vi "Calculate Dispersion.vi"(5 "grating index (current)":i8=-1, 7 "turret index (0)":u8, 8 "error in (no error)":errorcluster, 10 "wavelength, nm (current)":dbl=-1.0, 11 "SOL MS in":refnum<class "PL SOL Instruments MS.lvclass">) -> (0 "error out":errorcluster, 2 "dispersion, nm/mm":dbl, 3 "SOL MS out":refnum<class "PL SOL Instruments MS.lvclass">)   [LabVIEW 2015, in "PL SOL Instruments MS.lvclass"]
doc: "Calculates <b>dispersion</b> at the specified <b>wavelength</b> for the specified <b>grating</b> of the specified <b>turret</b>."
uses:
  PL SOL Instruments MS.lvclass
  PL SOL Instruments MS.lvclass/PL SOL Instruments MS.ctl
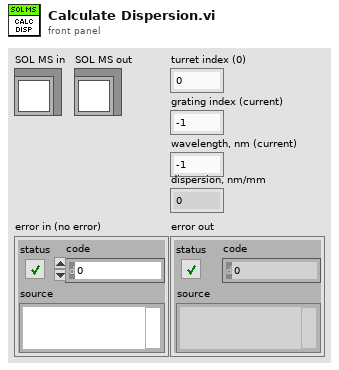
[diagram p1: front panel]
types:
  T1 = cluster{"name":string, "step timeout, ms":u32, "reset timeout, ms":u32, "gratings":cluster{"name":string, "step timeout, ms":u32, "reset timeout, ms":u32, "turret position":i32, "reset position":i32, "max position":i32, "backlash distance":i32, "step size, rad":dbl, "groove density, g/mm":dbl, "theta2, rad":dbl, "blaze wavelength, nm":dbl, "focal length, cm":dbl, "manual change":bool, "manual change position":i32}[], "current grating":cluster{"index":u8, "position":i32}}[]
  T2 = cluster{"name":string, "step timeout, ms":u32, "reset timeout, ms":u32, "gratings":cluster{"name":string, "step timeout, ms":u32, "reset timeout, ms":u32, "turret position":i32, "reset position":i32, "max position":i32, "backlash distance":i32, "step size, rad":dbl, "groove density, g/mm":dbl, "theta2, rad":dbl, "blaze wavelength, nm":dbl, "focal length, cm":dbl, "manual change":bool, "manual change position":i32}[], "current grating":cluster{"index":u8, "position":i32}}
  T3 = cluster{"name":string, "step timeout, ms":u32, "reset timeout, ms":u32, "turret position":i32, "reset position":i32, "max position":i32, "backlash distance":i32, "step size, rad":dbl, "groove density, g/mm":dbl, "theta2, rad":dbl, "blaze wavelength, nm":dbl, "focal length, cm":dbl, "manual change":bool, "manual change position":i32}[]
  T4 = cluster{"name":string, "step timeout, ms":u32, "reset timeout, ms":u32, "turret position":i32, "reset position":i32, "max position":i32, "backlash distance":i32, "step size, rad":dbl, "groove density, g/mm":dbl, "theta2, rad":dbl, "blaze wavelength, nm":dbl, "focal length, cm":dbl, "manual change":bool, "manual change position":i32}
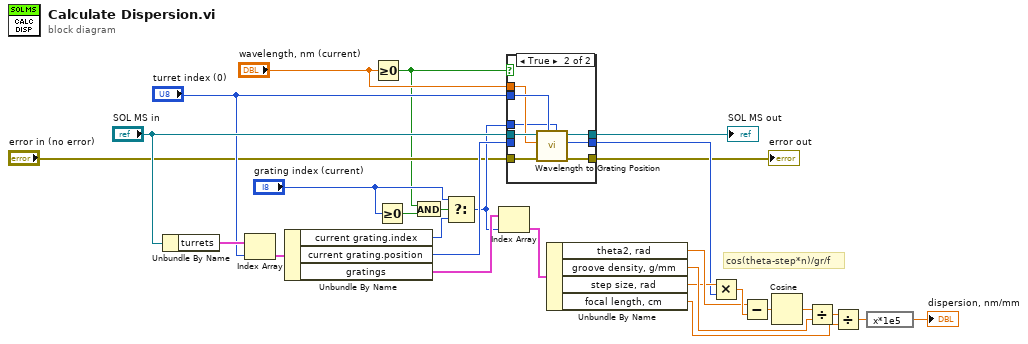
[diagram p0: block diagram]
diagram:
  # "cos(theta-step*n)/gr/f"
  n1 = Unbundle By Name("SOL MS in") -> ("turrets"=w25:T1)
  n2 = Index Array(array=w25, index="turret index (0)") -> (element=w13:T2)
  n3 = Unbundle By Name(w13) -> ("current grating.index"=w8:u8, "current grating.position"=w12:i32, "gratings"=w14:T3)
  n4 = Greater Or Equal To 0?(x="wavelength, nm (current)") -> (x >= 0?=w2:bool)
  n5 = Greater Or Equal To 0?(x="grating index (current)") -> (x >= 0?=w4:bool)
  n6 = And(x=w2, y=w4) -> (x .and. y?=w5:bool)
  n7 = Select(t="grating index (current)", s=w5, f=w8) -> (s? t:f=w7:u8)
  n8 = Index Array(array=w14, index=w7) -> (element=w15:T4)
  n9 = case shown="True" w2 {
    tunnel: "SOL MS in" -> [w31 w38]
    tunnel: [w31 w39] -> w27
    tunnel: "turret index (0)" -> [_ w37]
    tunnel: w12 -> [w30 _]
    tunnel: "wavelength, nm (current)" -> [_ w36]
    tunnel: [w30 w35] -> w11
    tunnel: w7 -> [_ w34]
    tunnel: "error in (no error)" -> [w29 w33]
    tunnel: [w29 w32] -> w1
    frame False {
    }
    frame True {
      n10 = call "Wavelength to Grating Position.vi"("grating index (0)"=w34, "turret index (0)"=w37, "error in (no error)"=w33, "wavelength, nm"=w36, "SOL MS in"=w38) -> ("error out"=w32:errorcluster, "grating position"=w35:i32, "SOL MS out"=w39:refnum<class "PL SOL Instruments MS.lvclass">)  [unwired: 4 in]
    }
  }
  "SOL MS out" <- w27
  "error out" <- w1
  n11 = Unbundle By Name(w15) -> ("theta2, rad"=w21:dbl, "groove density, g/mm"=w23:dbl, "step size, rad"=w16:dbl, "focal length, cm"=w24:dbl)
  n12 = Multiply(x=w16, y=w11) -> (x*y=w22:dbl)
  n13 = Subtract(x=w21, y=w22) -> (x-y=w17:dbl)
  n14 = Cosine(x=w17) -> (cos(x)=w18:dbl)
  n15 = Divide(x=w18, y=w23) -> (x/y=w19:dbl)
  n16 = Divide(x=w19, y=w24) -> (x/y=w20:dbl)
  n17 = expression code="x*1e5"(w20) -> (→"dispersion, nm/mm":dbl)
